vi "DSF.Engine.Memory.ObjectPool.Bundle.Set Object.vi"(8 "error in (no error)":errorcluster, 10 "Object":refnum<class>, 11 "ObjectPool Bundle in":refnum<class "DSF.Engine.Memory.ObjectPool.Bundle.lvclass">) -> (0 "error out":errorcluster, 3 "ObjectPool Bundle out":refnum<class "DSF.Engine.Memory.ObjectPool.Bundle.lvclass">)   [LabVIEW 2016, in "DSF.Engine.lvlib" / "DSF.Engine.Memory.ObjectPool.Bundle.lvclass"]
uses:
  DSF.Engine.Memory.ObjectPool.Bundle.lvclass
  DSF.Engine.Memory.ObjectPool.Bundle.lvclass/DSF.Engine.Memory.ObjectPool.Bundle.ctl
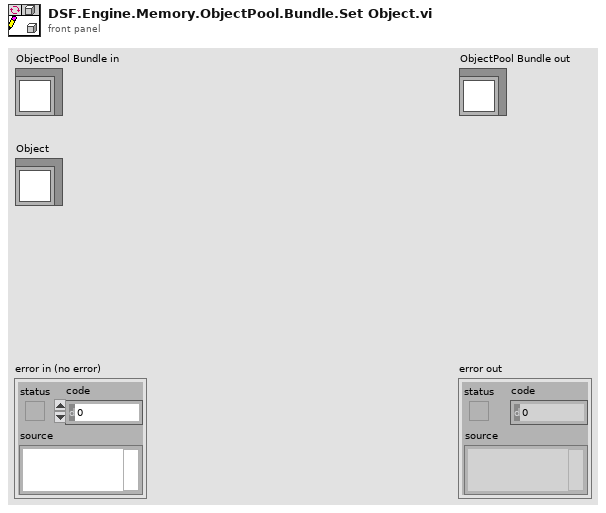
[diagram p1: front panel]
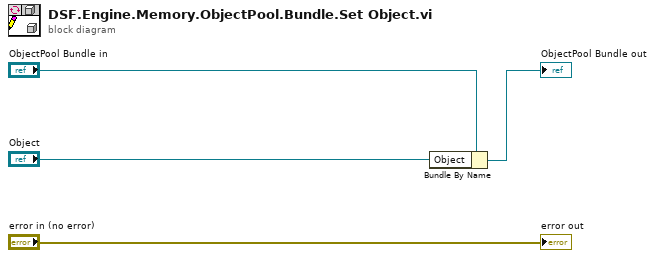
[diagram p0: block diagram]
diagram:
  n1 = Bundle By Name(cluster="ObjectPool Bundle in", "Object"="Object") -> (→"ObjectPool Bundle out":refnum<class "DSF.Engine.Memory.ObjectPool.Bundle.lvclass">)
  "error out" <- "error in (no error)"
